vi "calculate unit vector component.vi"(0 "event data at origin in":T1={"position [km]"=0.0, "time [nsec]"=20}, 7 "event data along axis in":T1={"position [km]"=384400.0, "time [nsec]"=365}, 11 "speed of light [m/s]":sgl=300000000.0) -> (8 "component of unit vector":sgl=-0.26925078)   [LabVIEW 2014]
doc: "This subVI calculates a component of a unit vector to a source along a given axis given the event data at the sensor along that axis, the event data at the origin, and the speed of light.\n\nPaul K Dixon\nP350\nCSUSB Physics\n\nBasic Algorithm:\n\ndefinitions:\nto = time at origin [nsec]\nta = time at sensor [nsec]\na = position of sensor along axis [m]\nv = speed of light [3E8 m/sec]\ndta = time interval from origin to sensor\nn = component of unit vector pointing to the source along the given axis [unitless]\n\ncalculations:\ndta = (ta-to)\nn = -(v*dta)/a"
uses:
  typedefs/event cluster typedef.ctl
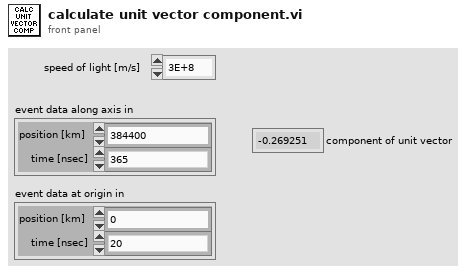
[diagram p1: front panel]
types:
  T1 = typedef "event cluster typedef.ctl" = cluster{"position [km]":sgl, "time [nsec]":i64}
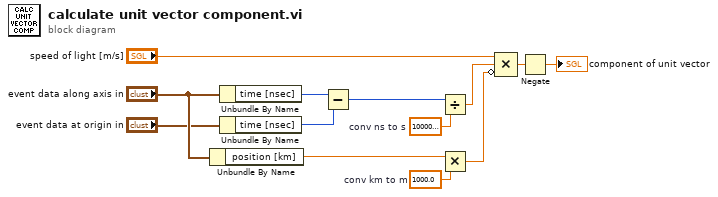
[diagram p0: block diagram]
diagram:
  w8 = sgl 1000.0  # conv km to m
  w5 = sgl 1000000000.0  # conv ns to s
  n1 = Unbundle By Name("event data along axis in") -> ("position [km]"=w7:sgl)
  n2 = Unbundle By Name("event data along axis in") -> ("time [nsec]"=w2:i64)
  n3 = Unbundle By Name("event data at origin in") -> ("time [nsec]"=w3:i64)
  n4 = Subtract(x=w2, y=w3) -> (x-y=w4:i64)
  n5 = Divide(x=w4, y=w5) -> (x/y=w10:sgl)
  n6 = Multiply(x=w7, y=w8) -> (x*y=w11:sgl)
  n7 = Compound Arithmetic op=MULTIPLY("speed of light [m/s]", w10, invert w11) -> (w12:sgl)
  n8 = Negate(x=w12) -> (-x=→"component of unit vector":sgl)
